vi "Periodic Tasks.vi"(8 "error in":errorcluster) -> ()   [LabVIEW 2020]
doc: "This VI runs in parallel to other tasks. It can contain as many user-defined periodic loops as you need. These can carry out PID or other sorts of timed response."
uses:
  Robot Global Data.vi
  <vilib>/Rock Robotics/Network Tables/NT Write Boolean.vi
  <vilib>/Rock Robotics/Network Tables/NT Write Numeric Array.vi
  <vilib>/Rock Robotics/Network Tables/NT Write Boolean Array.vi
  <vilib>/Rock Robotics/WPI/ThirdParty/Phoenix-LabVIEW/Motor Controller/Controls/CTRE_Phoenix_MotorControl_ControlMode.ctl
  <vilib>/Rock Robotics/WPI/DriverStation/WPI_DriverStationRobotMode2.ctl
  <vilib>/Rock Robotics/Network Tables/NT Write Number.vi
  <vilib>/Rock Robotics/WPI/RobotDrive/WPI_RobotDriveMecanumDrive_Cartesian.vi
  <vilib>/Rock Robotics/WPI/ThirdParty/Phoenix-LabVIEW/Motor Controller/Get/CTRE_Phoenix_MotorController_GetQuadratureData.vi
panel:
  out "Encoder":dbl
  out "Encoder Position":dbl
  out "Slow Speed ON":bool
  out "Backwards ON":bool
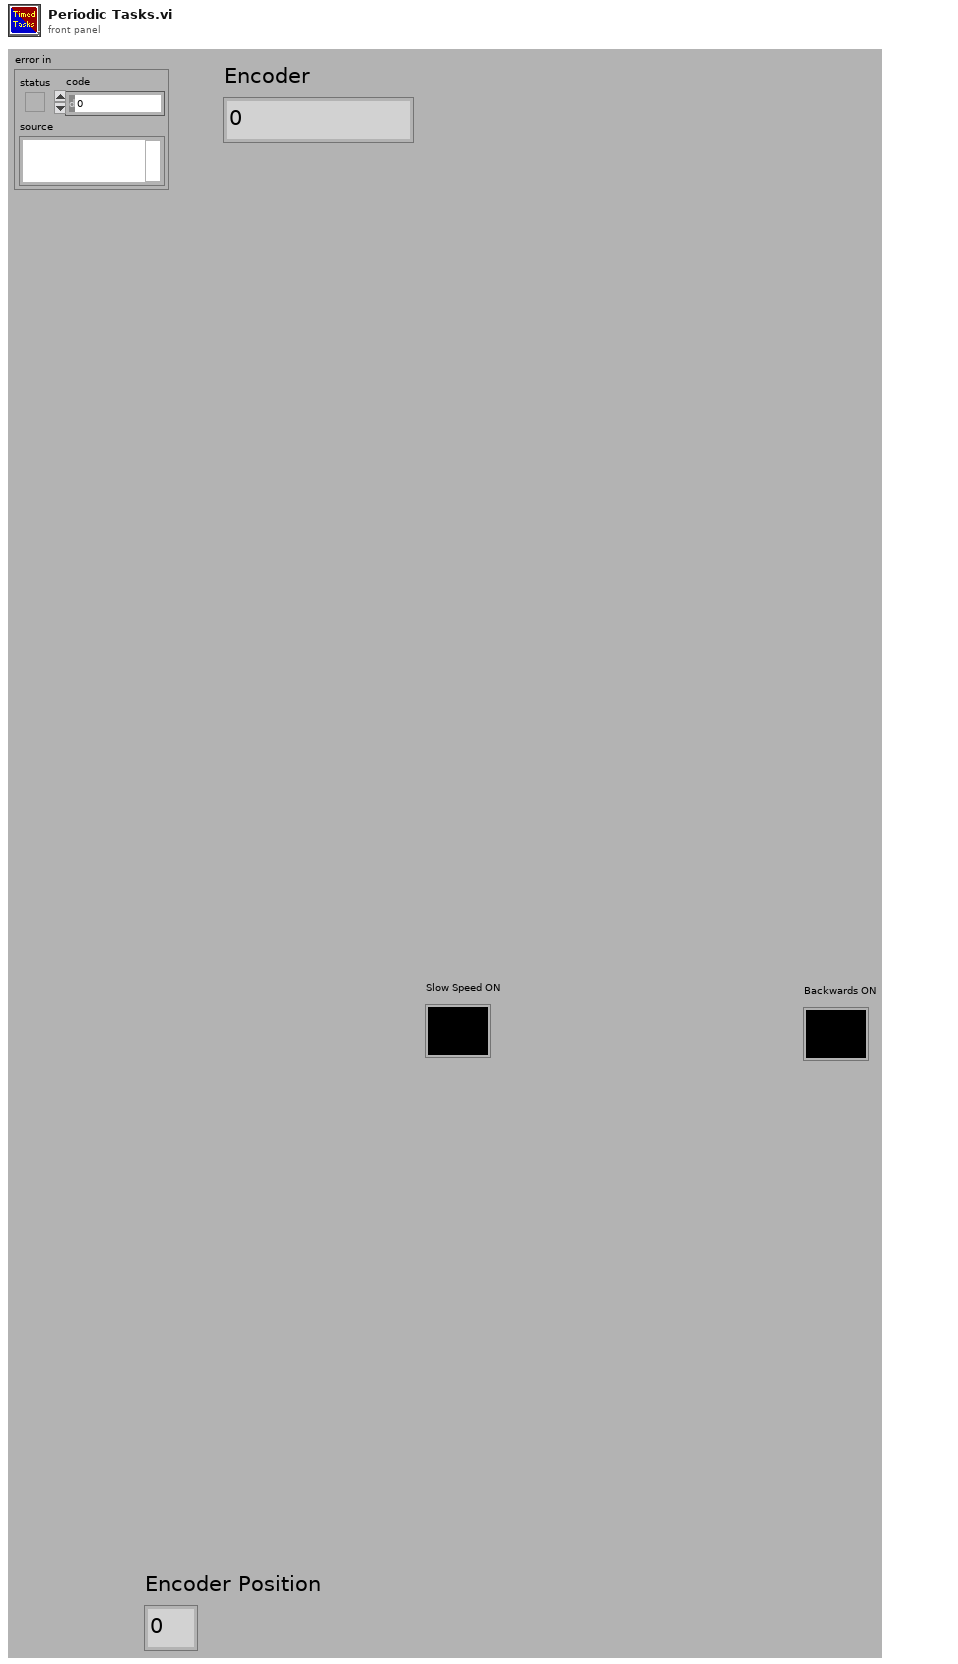
[diagram p1: front panel]
types:
  T1 = typedef "WPI_MotorControlDeviceRef.ctl" = cluster{"DeviceStatus":errorcluster, "Type":T2, "PWM":cluster{"PWM Channel":T3, "DeadBand":T4}, "CAN":cluster{"Device Number":u8, "SetOutput VI Ref":variant, "GetOutput VI Ref":variant, "Enable VI Ref":variant, "Disable VI Ref":variant, "Data":variant}, "Invert":bool, "DIO PWM":cluster{"PWM \"Enable\" Channel":T3, "DIOChannel":T5, "PWM Rate":dbl}}
  T2 = typedef "WPI_MotorControlType.ctl" = enum16{"PWM", "CAN", "DIO PWM"}
  T3 = typedef "FPGA_DIOPWMChannel.ctl" = enum8{"PWM 0", "PWM 1", "PWM 2", "PWM 3", "PWM 4", "PWM 5", "PWM 6", "PWM 7", "PWM 8", "PWM 9", "PWM MXP 0", "PWM MXP 1", "PWM MXP 2", "PWM MXP 3", "PWM MXP 4", "PWM MXP 5", "PWM MXP 6", "PWM MXP 7", "PWM MXP 8", "PWM MXP 9", "Invalid"}
  T4 = typedef "WPI_PWMDeadband.ctl" = cluster{"Name":string, "maxPositivePwm":i32, "minPositivePwm":i32, "centerPwm":i32, "maxNegativePwm":i32, "minNegativePwm":i32, "angularRange":u16}
  T5 = typedef "FPGA_DIOChannel.ctl" = enum8{"DIO 0", "DIO 1", "DIO 2", "DIO 3", "DIO 4", "DIO 5", "DIO 6", "DIO 7", "DIO 8", "DIO 9", "DIO MXP 0", "DIO MXP 1", "DIO MXP 2", "DIO MXP 3", "DIO MXP 4", "DIO MXP 5", "DIO MXP 6", "DIO MXP 7", "DIO MXP 8", "DIO MXP 9", "DIO MXP 10", "DIO MXP 11", "DIO MXP 12", "DIO MXP 13", "DIO MXP 14", "DIO MXP 15", "SPI Port CS1", "SPI Port CS2", "SPI Port CS3", "SPI Port MISO", "SPI Port MOSI", "Invalid"}
  T6 = typedef "WPI_JoystickDevRef.ctl" = cluster{"Device":T7}
  T7 = typedef "WPI_JoystickDeviceEnum.ctl" = enum16{"USB 0", "USB 1", "USB 2", "USB 3", "USB 4", "USB 5"}
  T8 = typedef "WPI_RobotDriveDevRef.ctl" = cluster{"DevStatus":errorcluster, "Motors[]":T1[], "Square Inputs":bool, "Max Output":dbl}
  T9 = typedef "WPI_ServoDeviceRef.ctl" = cluster{"DeviceStatus":errorcluster, "PWM Channel":T3, "DeadBand":T4}
  T10 = typedef "WPI_DriverStationRobotMode2.ctl" = enum16{"Autonomous Disabled", "Autonomous Enabled", "Teleop Disabled", "Teleop Enabled", "Disconnected", "Finish", "Test Disabled", "Test Enabled", "Emergency Stopped"}
  T11 = typedef "CTRE_Phoenix_MotorControl_ControlMode.ctl" = u16
  T12 = typedef "WPI_GyroDevRef.ctl" = cluster{"DevStatus":errorcluster, "Analog Channel":T13, "Gain (VoltsPerDegree/Second)":dbl, "Gyro Type":enum16{"Analog", "XRS450"}, "Handle":i32, "SPI Bus":T14, "Device Found":bool, "Sample Rate":dbl, "Calibrate On Open":bool, "Offset":dbl}
  T13 = typedef "FPGA_AIChannel.ctl" = enum8{"AI 0", "AI 1", "AI 2", "AI 3", "AI MXP 0", "AI MXP 1", "AI MXP 2", "AI MXP 3", "Invalid"}
  T14 = typedef "spi_bus.ctl" = enum16{"SPI On-Board, CS0", "SPI On-Board, CS1", "SPI On-Board, CS2", "SPI On-Board, CS3", "SPI MXP", "Invalid"}
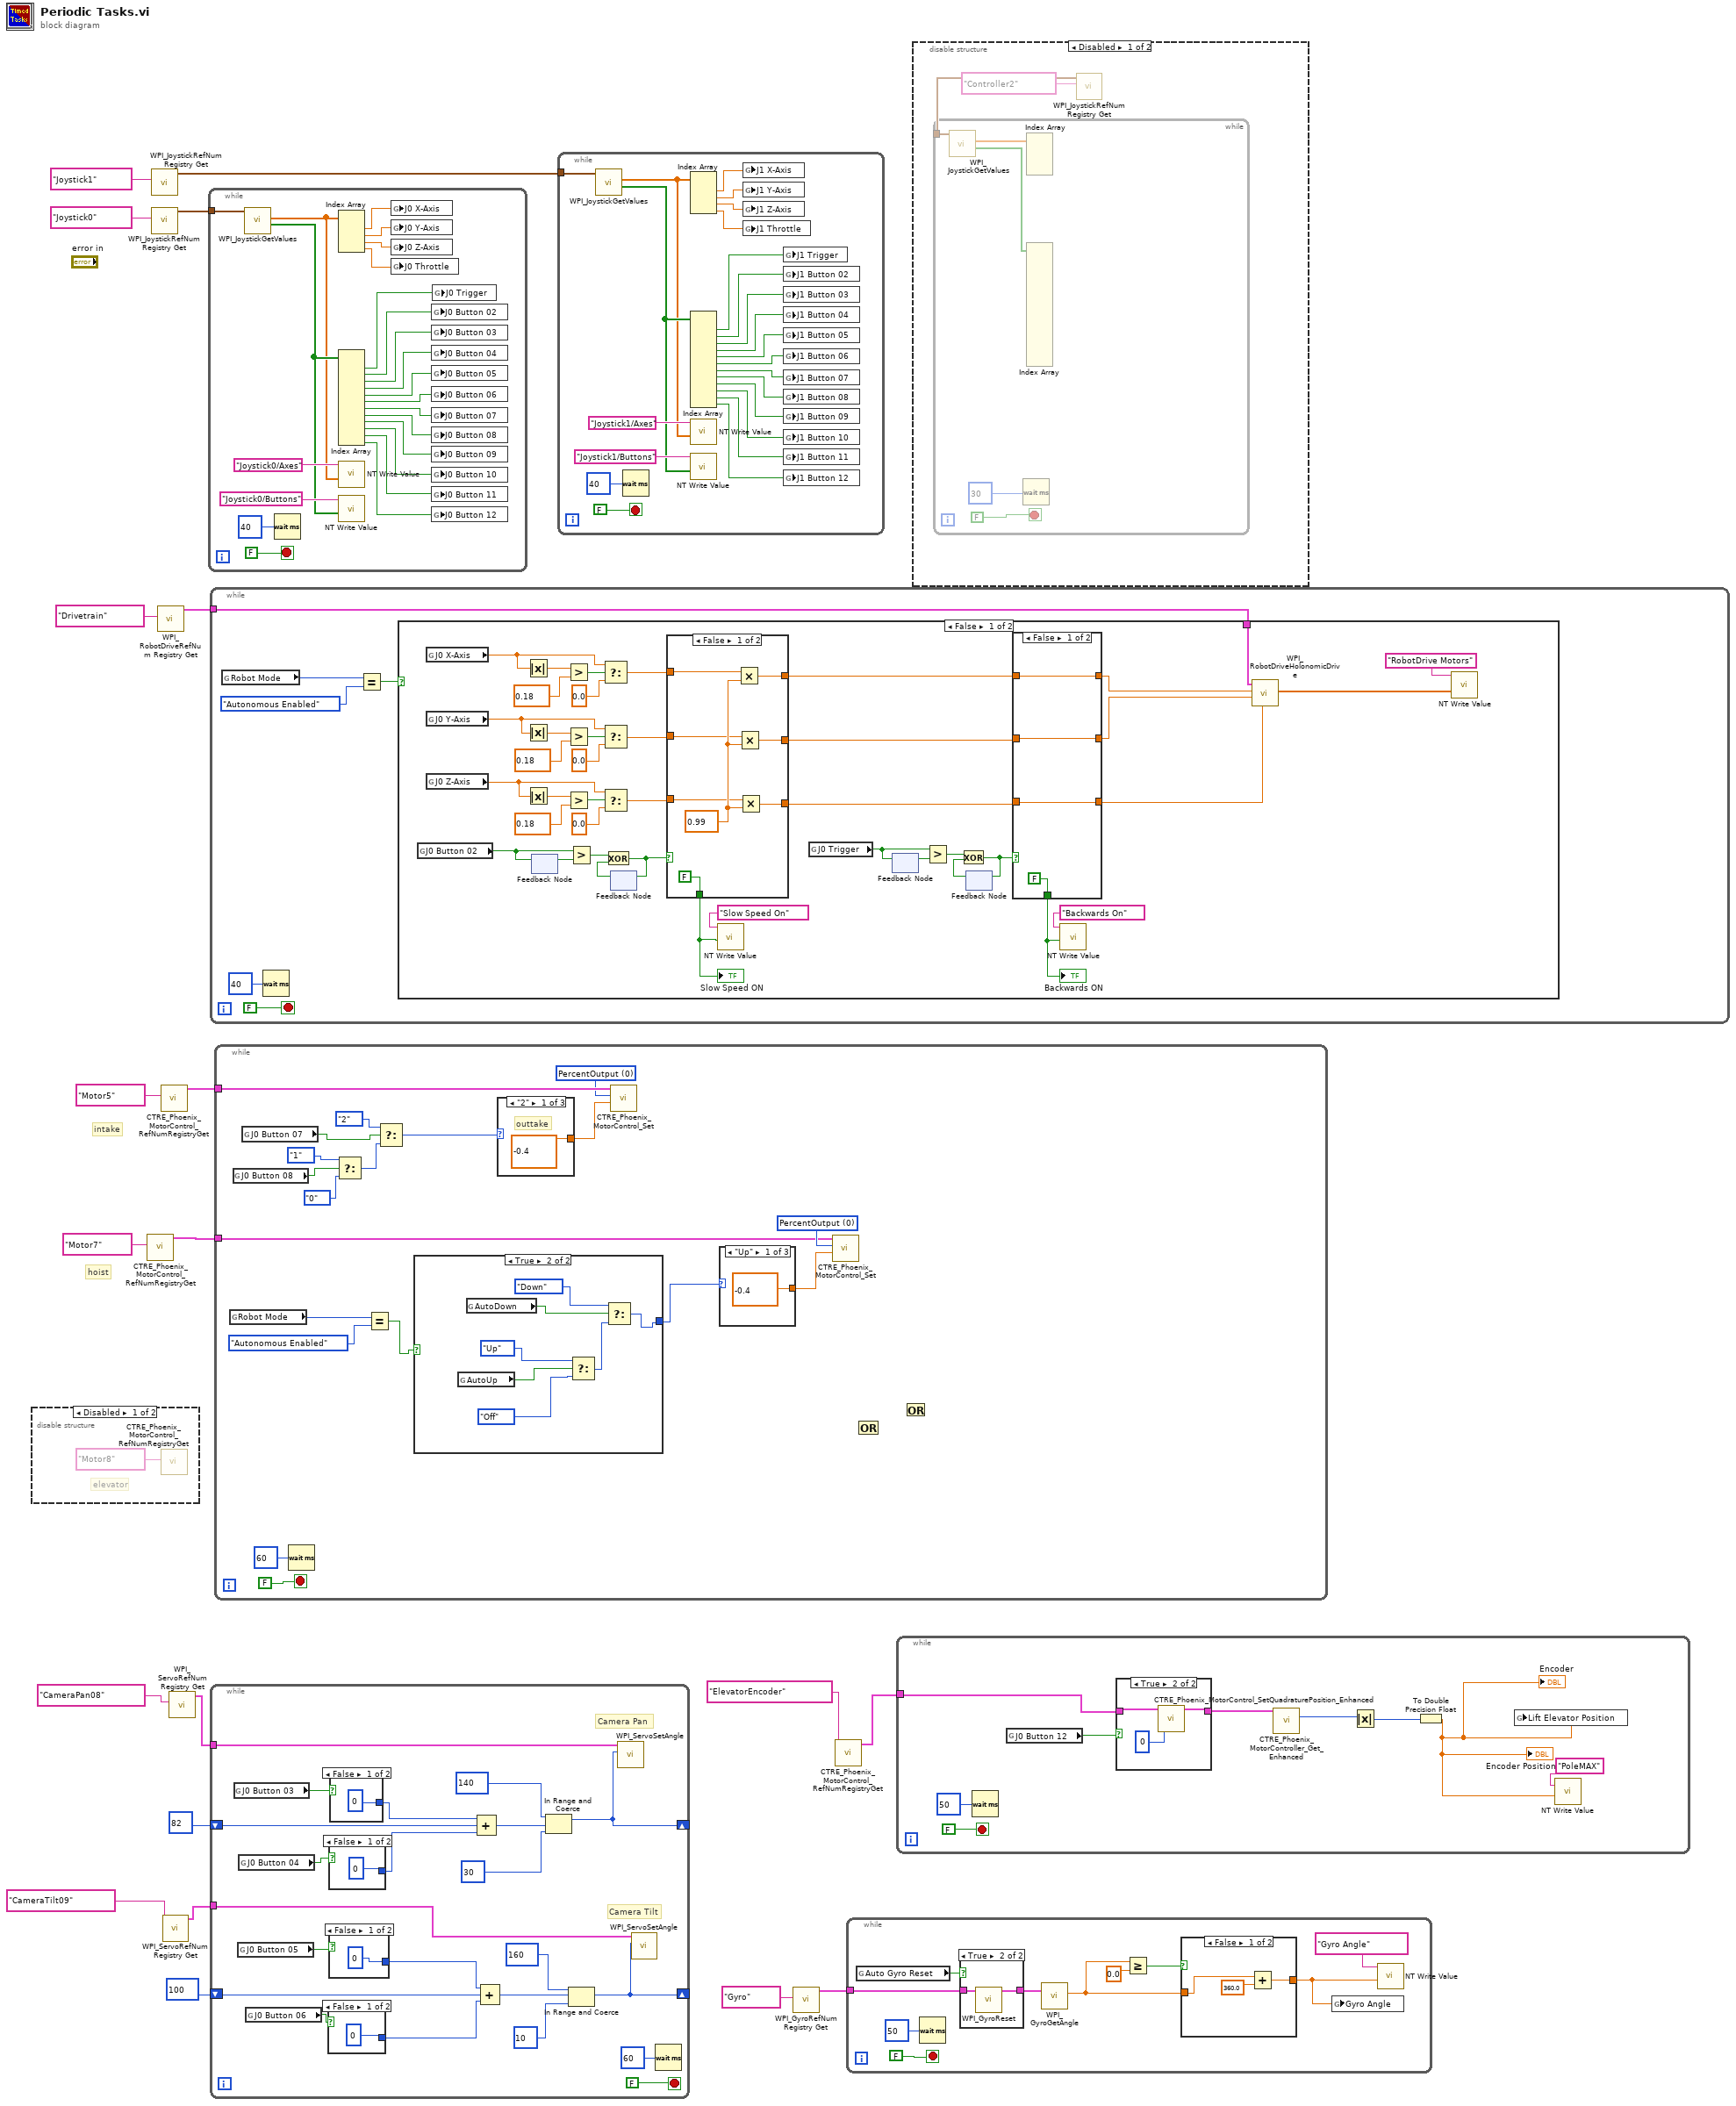
[diagram p0: block diagram]
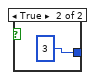
[diagram p6: hidden frame]
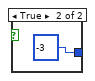
[diagram p7: hidden frame]
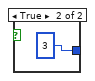
[diagram p8: hidden frame]
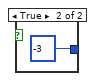
[diagram p9: hidden frame]
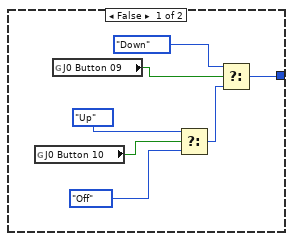
[diagram p11: hidden frame]
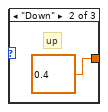
[diagram p12: hidden frame]
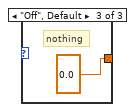
[diagram p13: hidden frame]
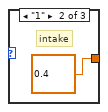
[diagram p14: hidden frame]
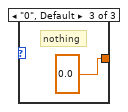
[diagram p15: hidden frame]
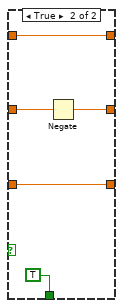
[diagram p16: hidden frame]
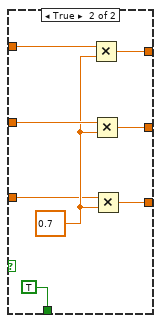
[diagram p17: hidden frame]
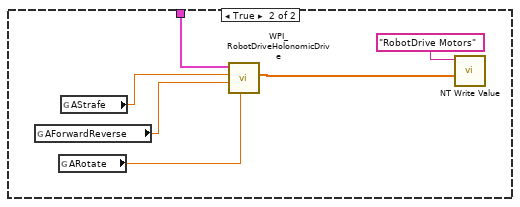
[diagram p18: hidden frame]
diagram:
  # "hoist"
  # "intake"
  n1 = disable-structure shown="Disabled" {
    frame Disabled {
      # "elevator"
      n2 = call <vilib>:"CTRE_Phoenix_MotorControl_RefNumRegistryGet.vi"("refnum name"="Motor8") -> ()  [unwired: 9 in, 2 out]
    }
    frame Enabled {
    }
  }
  n3 = call <vilib>:"CTRE_Phoenix_MotorControl_RefNumRegistryGet.vi"("refnum name"="Motor7") -> ("PhoenixMotorControlDevRef"=w12:T1)  [unwired: 9 in, 1 out]
  n4 = call <vilib>:"WPI_JoystickRefNum Registry Get.vi"("refnum name"="Joystick1") -> ("JoystickDevRef"=w16:T6)  [unwired: 1 in, 9 out]
  n5 = call <vilib>:"WPI_JoystickRefNum Registry Get.vi"("refnum name"="Joystick0") -> ("JoystickDevRef"=w18:T6)  [unwired: 1 in, 9 out]
  n6 = call <vilib>:"WPI_RobotDriveRefNum Registry Get.vi"("refnum name"="Drivetrain") -> ("RobotDriveDevRef"=w3:T8)  [unwired: 9 in, 1 out]
  n7 = call <vilib>:"CTRE_Phoenix_MotorControl_RefNumRegistryGet.vi"("refnum name"="Motor5") -> ("PhoenixMotorControlDevRef"=w13:T1)  [unwired: 9 in, 1 out]
  n8 = call <vilib>:"WPI_ServoRefNum Registry Get.vi"("refnum name"="CameraTilt09") -> ("ServoDeviceRef"=w8:T9)  [unwired: 9 in, 1 out]
  n9 = call <vilib>:"WPI_ServoRefNum Registry Get.vi"("refnum name"="CameraPan08") -> ("ServoDeviceRef"=w9:T9)  [unwired: 9 in, 1 out]
  n10 = while {
    tunnel: w18 -> [w42]
    stop <- FALSE stop-if-true
    n11 = call <vilib>:"WPI_JoystickGetValues.vi"("JoystickDevRef"=w42) -> ("Buttons"=w23:bool[], "Axes"=w22:dbl[])  [unwired: 6 in, 3 out]
    n12 = Wait (ms)(milliseconds to wait=u32 40) -> ()  [unwired: 1 out]
    n13 = Index Array(array=w22) -> (element #1=w41:dbl, element #2=w40:dbl, element #3=w39:dbl, element #4=w38:dbl)  [unwired: 4 in]
    n14 = Index Array(array=w23) -> (element #1=w37:bool, element #2=w36:bool, element #3=w35:bool, element #4=w34:bool, element #5=w33:bool, element #6=w32:bool, element #7=w31:bool, element #8=w30:bool, element #9=w29:bool, element #10=w28:bool, element #11=w27:bool, element #12=w26:bool)  [unwired: 12 in]
    n15 = call-poly <vilib>:"NT Write Value.vi"("Numeric Array"=w22, "Name"="Joystick0/Axes") -> ()  [unwired: 9 in, 1 out]
    n16 = call-poly <vilib>:"NT Write Value.vi"("Boolean Array"=w23, "Name"="Joystick0/Buttons") -> ()  [unwired: 9 in, 1 out]
    n17 = global write "Robot Global Data.vi" "J0 X-Axis"(w41) -> ()
    n18 = global write "Robot Global Data.vi" "J0 Y-Axis"(w40) -> ()
    n19 = global write "Robot Global Data.vi" "J0 Z-Axis"(w39) -> ()
    n20 = global write "Robot Global Data.vi" "J0 Throttle"(w38) -> ()
    n21 = global write "Robot Global Data.vi" "J0 Button 02"(w36) -> ()
    n22 = global write "Robot Global Data.vi" "J0 Button 03"(w35) -> ()
    n23 = global write "Robot Global Data.vi" "J0 Button 04"(w34) -> ()
    n24 = global write "Robot Global Data.vi" "J0 Button 05"(w33) -> ()
    n25 = global write "Robot Global Data.vi" "J0 Button 06"(w32) -> ()
    n26 = global write "Robot Global Data.vi" "J0 Button 07"(w31) -> ()
    n27 = global write "Robot Global Data.vi" "J0 Button 08"(w30) -> ()
    n28 = global write "Robot Global Data.vi" "J0 Button 09"(w29) -> ()
    n29 = global write "Robot Global Data.vi" "J0 Button 10"(w28) -> ()
    n30 = global write "Robot Global Data.vi" "J0 Button 11"(w27) -> ()
    n31 = global write "Robot Global Data.vi" "J0 Button 12"(w26) -> ()
    n32 = global write "Robot Global Data.vi" "J0 Trigger"(w37) -> ()
  }
  n33 = while {
    tunnel: w3 -> [w45]
    stop <- FALSE stop-if-true
    n34 = global read "Robot Global Data.vi" "Robot Mode"() -> (w48:T10)
    n35 = Wait (ms)(milliseconds to wait=u32 40) -> ()  [unwired: 1 out]
    n36 = Equal?(x=w48, y=WPI_DriverStationRobotMode2."Autonomous Enabled" ("Robot Mode")) -> (x = y?=w46:bool)
    n37 = case shown="False" w46 {
      tunnel: w45 -> [w53 w122]
      frame False {
        n38 = global read "Robot Global Data.vi" "J0 Button 02"() -> (w66:bool)
        n39 = global read "Robot Global Data.vi" "J0 X-Axis"() -> (w70:dbl)
        n40 = global read "Robot Global Data.vi" "J0 Y-Axis"() -> (w69:dbl)
        n41 = global read "Robot Global Data.vi" "J0 Z-Axis"() -> (w68:dbl)
        n42 = Absolute Value(x=w70) -> (abs(x)=w85:dbl)
        n43 = Absolute Value(x=w69) -> (abs(x)=w87:dbl)
        n44 = Absolute Value(x=w68) -> (abs(x)=w79:dbl)
        n45 = feedback #1() -> (w90:bool)  [unwired: 1 in]
        n46 = feedback-in #1(w66) -> ()
        n47 = Greater?(x=w85, y=0.18) -> (0:w86:bool)
        n48 = Greater?(x=w87, y=0.18) -> (0:w88:bool)
        n49 = Greater?(x=w79, y=0.18) -> (0:w80:bool)
        n50 = Greater?(x=w66, y=w90) -> (0:w89:bool)
        n51 = Select(t=w70, s=w86, f=0.0) -> (s? t:f=w71:dbl)
        n52 = Select(t=w69, s=w88, f=0.0) -> (s? t:f=w72:dbl)
        n53 = Select(t=w68, s=w80, f=0.0) -> (s? t:f=w73:dbl)
        n54 = feedback #2() -> (w91:bool)  [unwired: 1 in]
        n55 = Exclusive Or(1:w91, 2:w89) -> (0:w67:bool)
        n56 = feedback-in #2(w67) -> ()
        n57 = case shown="False" w67 {
          tunnel: w71 -> [w107 w116]
          tunnel: w72 -> [w106 w115]
          tunnel: [w104 w114] -> w59
          tunnel: [w103 w113] -> w58
          tunnel: w73 -> [w105 w111]
          tunnel: [w102 w110] -> w57
          tunnel: [FALSE ("Boolean") TRUE ("Boolean")] -> w65
          frame False {
            w108 = 0.99 ("y")
            n58 = Multiply(x=w107, y=w108) -> (x*y=w104:dbl)
            n59 = Multiply(x=w106, y=w108) -> (x*y=w103:dbl)
            n60 = Multiply(x=w105, y=w108) -> (x*y=w102:dbl)
          }
          frame True {
            w112 = 0.7 ("y")
            n61 = Multiply(x=w116, y=w112) -> (x*y=w114:dbl)
            n62 = Multiply(x=w115, y=w112) -> (x*y=w113:dbl)
            n63 = Multiply(x=w111, y=w112) -> (x*y=w110:dbl)
          }
        }
        "Slow Speed ON" <- w65
        n64 = call-poly <vilib>:"NT Write Value.vi"("Boolean"=w65, "Name"="Slow Speed On") -> ()  [unwired: 9 in, 1 out]
        n65 = global read "Robot Global Data.vi" "J0 Trigger"() -> (w64:bool)
        n66 = feedback #3() -> (w63:bool)  [unwired: 1 in]
        n67 = feedback-in #3(w64) -> ()
        n68 = Greater?(x=w64, y=w63) -> (0:w74:bool)
        n69 = feedback #4() -> (w62:bool)  [unwired: 1 in]
        n70 = Exclusive Or(1:w62, 2:w74) -> (0:w61:bool)
        n71 = feedback-in #4(w61) -> ()
        n72 = case shown="False" w61 {
          tunnel: w58 -> [w94 w99]
          tunnel: w59 -> [w92 w97]
          tunnel: [w94 w98] -> w55
          tunnel: [w92 w97] -> w54
          tunnel: w57 -> [w93 w96]
          tunnel: [w93 w96] -> w56
          tunnel: [FALSE ("Boolean") TRUE ("Boolean")] -> w60
          frame False {
          }
          frame True {
            n73 = Negate(x=w99) -> (-x=w98:dbl)
          }
        }
        "Backwards ON" <- w60
        n74 = call-poly <vilib>:"NT Write Value.vi"("Boolean"=w60, "Name"="Backwards On") -> ()  [unwired: 9 in, 1 out]
        n75 = call-poly <vilib>:"WPI_RobotDriveHolonomicDrive.vi"("Rotation"=w56, "Y"=w55, "X"=w54, "RobotDriveDevRef"=w53) -> ("Motor Values"=w51:dbl[])  [unwired: 5 in, 2 out]
        n76 = call-poly <vilib>:"NT Write Value.vi"("Numeric Array"=w51, "Name"="RobotDrive Motors") -> ()  [unwired: 9 in, 1 out]
      }
      frame True {
        n77 = global read "Robot Global Data.vi" "AForwardReverse"() -> (w119:dbl)
        n78 = global read "Robot Global Data.vi" "ARotate"() -> (w121:dbl)
        n79 = global read "Robot Global Data.vi" "AStrafe"() -> (w120:dbl)
        n80 = call-poly <vilib>:"WPI_RobotDriveHolonomicDrive.vi"("Rotation"=w121, "Y"=w119, "X"=w120, "RobotDriveDevRef"=w122) -> ("Motor Values"=w118:dbl[])  [unwired: 5 in, 2 out]
        n81 = call-poly <vilib>:"NT Write Value.vi"("Numeric Array"=w118, "Name"="RobotDrive Motors") -> ()  [unwired: 9 in, 1 out]
      }
    }
  }
  n82 = while {
    tunnel: w9 -> [w144]
    tunnel: w8 -> [w143]
    shift-right: [w131] -> _
    shift-left: 82 -> [w124]
    shift-right: [w123] -> _
    shift-left: 100 -> [w140]
    stop <- FALSE stop-if-true
    # "Camera Tilt"
    # "Camera Pan"
    n83 = global read "Robot Global Data.vi" "J0 Button 03"() -> (w127:bool)
    n84 = global read "Robot Global Data.vi" "J0 Button 05"() -> (w129:bool)
    n85 = global read "Robot Global Data.vi" "J0 Button 04"() -> (w128:bool)
    n86 = global read "Robot Global Data.vi" "J0 Button 06"() -> (w130:bool)
    n87 = case shown="False" w130 {
      tunnel: [0 3] -> w139
      frame False {
      }
      frame True {
      }
    }
    n88 = case shown="False" w128 {
      tunnel: [0 3] -> w141
      frame False {
      }
      frame True {
      }
    }
    n89 = case shown="False" w129 {
      tunnel: [0 -3] -> w138
      frame False {
      }
      frame True {
      }
    }
    n90 = case shown="False" w127 {
      tunnel: [0 -3] -> w142
      frame False {
      }
      frame True {
      }
    }
    n91 = Compound Arithmetic op=ADD(w142, w124, w141) -> (w135:i32)
    n92 = Compound Arithmetic op=ADD(w138, w140, w139) -> (w132:i32)
    n93 = In Range and Coerce(upper limit=140, x=w135, lower limit=30) -> (coerced(x)=w131:i32)  [unwired: 1 out]
    n94 = In Range and Coerce(upper limit=160, x=w132, lower limit=10) -> (coerced(x)=w123:i32)  [unwired: 1 out]
    n95 = call <vilib>:"WPI_ServoSetAngle.vi"("Angle"=w131, "ServoDeviceRef"=w144) -> ()  [unwired: 8 in, 2 out]
    n96 = call <vilib>:"WPI_ServoSetAngle.vi"("Angle"=w123, "ServoDeviceRef"=w143) -> ()  [unwired: 8 in, 2 out]
    n97 = Wait (ms)(milliseconds to wait=u32 60) -> ()  [unwired: 1 out]
  }
  n98 = while {
    tunnel: w13 -> [w171]
    tunnel: w12 -> [w157]
    stop <- FALSE stop-if-true
    w160 = T11 0 items=["PercentOutput"=0, "Position"=1, "Velocity"=2, "Current"=3, "Follower"=5, "MotionProfile"=6, "MotionMagic"=7, "MotionProfileArc"=10, "Disabled"=15] ("Control Mode")
    w170 = T11 0 items=["PercentOutput"=0, "Position"=1, "Velocity"=2, "Current"=3, "Follower"=5, "MotionProfile"=6, "MotionMagic"=7, "MotionProfileArc"=10, "Disabled"=15] ("Control Mode")
    n99 = global read "Robot Global Data.vi" "Robot Mode"() -> (w155:T10)
    n100 = global read "Robot Global Data.vi" "J0 Button 08"() -> (w156:bool)
    n101 = global read "Robot Global Data.vi" "J0 Button 07"() -> (w165:bool)
    n102 = Wait (ms)(milliseconds to wait=u32 60) -> ()  [unwired: 1 out]
    n103 = Select(t=enum16{"2", "1", "0", ""}."1", s=w156, f=enum16{"2", "1", "0", ""}."0") -> (s? t:f=w166:enum16{"2", "1", "0", ""})
    n104 = Equal?(x=w155, y=WPI_DriverStationRobotMode2."Autonomous Enabled" ("Robot Mode")) -> (x = y?=w153:bool)
    n105 = Select(t=enum16{"2", "1", "0", ""}."2", s=w165, f=w166) -> (s? t:f=w164:enum16{"2", "1", "0", ""})
    n106 = case shown="True" w153 {
      tunnel: [w176 w179] -> w158
      frame False {
        n107 = global read "Robot Global Data.vi" "J0 Button 10"() -> (w175:bool)
        n108 = global read "Robot Global Data.vi" "J0 Button 09"() -> (w177:bool)
        n109 = Select(t=enum16{"Up", "Down", "Off"}."Up", s=w175, f=enum16{"Up", "Down", "Off"}."Off") -> (s? t:f=w178:enum16{"Up", "Down", "Off"})
        n110 = Select(t=enum16{"Up", "Down", "Off"}."Down", s=w177, f=w178) -> (s? t:f=w176:enum16{"Up", "Down", "Off"})
      }
      frame True {
        n111 = global read "Robot Global Data.vi" "AutoUp"() -> (w185:bool)
        n112 = global read "Robot Global Data.vi" "AutoDown"() -> (w184:bool)
        n113 = Select(t=enum16{"Up", "Down", "Off"}."Up", s=w185, f=enum16{"Up", "Down", "Off"}."Off") -> (s? t:f=w183:enum16{"Up", "Down", "Off"})
        n114 = Select(t=enum16{"Up", "Down", "Off"}."Down", s=w184, f=w183) -> (s? t:f=w179:enum16{"Up", "Down", "Off"})
      }
    }
    n115 = case shown="\"2\"" w164 {
      tunnel: [-0.4 0.4 0.0] -> w169
      frame "2" {
        # "outtake"
      }
      frame "1" {
        # "intake"
      }
      frame "0", Default {
        # "nothing"
      }
    }
    n116 = call <vilib>:"CTRE_Phoenix_MotorControl_Set.vi"("Output"=w169, "Control Mode"=w170, "PhoenixMotorControlDevRef"=w171) -> ()  [unwired: 7 in, 2 out]
    n117 = case shown="\"Up\"" w158 {
      tunnel: [-0.4 0.4 0.0] -> w159
      frame "Up" {
      }
      frame "Down" {
        # "up"
      }
      frame "Off", Default {
        # "nothing"
      }
    }
    n118 = call <vilib>:"CTRE_Phoenix_MotorControl_Set.vi"("Output"=w159, "Control Mode"=w160, "PhoenixMotorControlDevRef"=w157) -> ()  [unwired: 7 in, 2 out]
    n119 = Compound Arithmetic op=OR() -> ()  [unwired: 2 in, 1 out]
    n120 = Or() -> ()  [unwired: 2 in, 1 out]
  }
  n121 = while {
    tunnel: w16 -> [w212]
    stop <- FALSE stop-if-true
    n122 = call <vilib>:"WPI_JoystickGetValues.vi"("JoystickDevRef"=w212) -> ("Buttons"=w193:bool[], "Axes"=w192:dbl[])  [unwired: 6 in, 3 out]
    n123 = Wait (ms)(milliseconds to wait=u32 40) -> ()  [unwired: 1 out]
    n124 = Index Array(array=w192) -> (element #1=w211:dbl, element #2=w210:dbl, element #3=w209:dbl, element #4=w208:dbl)  [unwired: 4 in]
    n125 = Index Array(array=w193) -> (element #1=w207:bool, element #2=w206:bool, element #3=w205:bool, element #4=w204:bool, element #5=w203:bool, element #6=w202:bool, element #7=w201:bool, element #8=w200:bool, element #9=w199:bool, element #10=w198:bool, element #11=w197:bool, element #12=w196:bool)  [unwired: 12 in]
    n126 = call-poly <vilib>:"NT Write Value.vi"("Numeric Array"=w192, "Name"="Joystick1/Axes") -> ()  [unwired: 9 in, 1 out]
    n127 = call-poly <vilib>:"NT Write Value.vi"("Boolean Array"=w193, "Name"="Joystick1/Buttons") -> ()  [unwired: 9 in, 1 out]
    n128 = global write "Robot Global Data.vi" "J1 X-Axis"(w211) -> ()
    n129 = global write "Robot Global Data.vi" "J1 Y-Axis"(w210) -> ()
    n130 = global write "Robot Global Data.vi" "J1 Z-Axis"(w209) -> ()
    n131 = global write "Robot Global Data.vi" "J1 Throttle"(w208) -> ()
    n132 = global write "Robot Global Data.vi" "J1 Trigger"(w207) -> ()
    n133 = global write "Robot Global Data.vi" "J1 Button 02"(w206) -> ()
    n134 = global write "Robot Global Data.vi" "J1 Button 03"(w205) -> ()
    n135 = global write "Robot Global Data.vi" "J1 Button 04"(w204) -> ()
    n136 = global write "Robot Global Data.vi" "J1 Button 05"(w203) -> ()
    n137 = global write "Robot Global Data.vi" "J1 Button 06"(w202) -> ()
    n138 = global write "Robot Global Data.vi" "J1 Button 07"(w201) -> ()
    n139 = global write "Robot Global Data.vi" "J1 Button 08"(w200) -> ()
    n140 = global write "Robot Global Data.vi" "J1 Button 09"(w199) -> ()
    n141 = global write "Robot Global Data.vi" "J1 Button 10"(w198) -> ()
    n142 = global write "Robot Global Data.vi" "J1 Button 11"(w197) -> ()
    n143 = global write "Robot Global Data.vi" "J1 Button 12"(w196) -> ()
  }
  n144 = call <vilib>:"WPI_GyroRefNum Registry Get.vi"("refnum name"="Gyro") -> ("GyroDevRef"=w6:T12)  [unwired: 9 in, 1 out]
  n145 = call <vilib>:"CTRE_Phoenix_MotorControl_RefNumRegistryGet.vi"("refnum name"="ElevatorEncoder") -> ("PhoenixMotorControlDevRef"=w1:T1)  [unwired: 9 in, 1 out]
  n146 = while {
    tunnel: w6 -> [w224]
    stop <- FALSE stop-if-true
    n147 = global read "Robot Global Data.vi" "Auto Gyro Reset"() -> (w222:bool)
    n148 = Wait (ms)(milliseconds to wait=u32 50) -> ()  [unwired: 1 out]
    n149 = case shown="True" w222 {
      tunnel: w224 -> [w229 w231]
      tunnel: [w229 w230] -> w223
      frame False {
      }
      frame True {
        n150 = call <vilib>:"WPI_GyroReset.vi"("GyroDevRef"=w231) -> ("GyroDevRef"=w230:T12)  [unwired: 9 in, 1 out]
      }
    }
    n151 = call <vilib>:"WPI_GyroGetAngle.vi"("GyroDevRef"=w223) -> ("Angle"=w219:dbl)  [unwired: 6 in, 4 out]
    n152 = Greater Or Equal?(x=w219, y=0.0) -> (x >= y?=w217:bool)
    n153 = case shown="False" w217 {
      tunnel: w219 -> [w226 w228]
      tunnel: [w225 w228] -> w215
      frame False {
        n154 = Add(x=w226, y=360.0) -> (x+y=w225:dbl)
      }
      frame True {
      }
    }
    n155 = global write "Robot Global Data.vi" "Gyro Angle"(w215) -> ()
    n156 = call-poly <vilib>:"NT Write Value.vi"("Numeric"=w215, "Name"="Gyro Angle" ("refnum name")) -> ()  [unwired: 9 in, 1 out]
  }
  n157 = while {
    tunnel: w1 -> [w238]
    stop <- FALSE stop-if-true
    n158 = Wait (ms)(milliseconds to wait=u32 50) -> ()  [unwired: 1 out]
    n159 = global read "Robot Global Data.vi" "J0 Button 12"() -> (w237:bool)
    n160 = case shown="True" w237 {
      tunnel: [w241 w243] -> w236
      tunnel: w238 -> [w241 w242]
      frame False {
      }
      frame True {
        n161 = call <vilib>:"CTRE_Phoenix_MotorControl_SetQuadraturePosition_Enhanced.vi"("New Position"=0, "PhoenixMotorControlDevRef"=w242) -> ("PhoenixMotorControlDevRef"=w243:T1)  [unwired: 8 in, 1 out]
      }
    }
    n162 = call-poly <vilib>:"CTRE_Phoenix_MotorController_Get_Enhanced.vi"("PhoenixMotorControlDevRef"=w236) -> ("Quadrature Position"=w235:i32)  [unwired: 11 in, 3 out]
    n163 = Absolute Value(x=w235) -> (abs(x)=w234:i32)
    n164 = To Double Precision Float(number=w234) -> (double precision float=w232:dbl)
    "Encoder Position" <- w232
    "Encoder" <- w232
    n165 = global write "Robot Global Data.vi" "Lift Elevator Position"(w232) -> ()
    n166 = call-poly <vilib>:"NT Write Value.vi"("Numeric"=w232, "Name"="PoleMAX") -> ()  [unwired: 9 in, 1 out]
  }
  n167 = disable-structure shown="Disabled" {
    frame Disabled {
      n168 = call <vilib>:"WPI_JoystickRefNum Registry Get.vi"("refnum name"="Controller2") -> ("JoystickDevRef"=w245:T6)  [unwired: 1 in, 9 out]
      n169 = while {
        tunnel: w245 -> [w251]
        stop <- FALSE stop-if-true
        n170 = call <vilib>:"WPI_JoystickGetValues.vi"("JoystickDevRef"=w251) -> ("Buttons"=w247:bool[], "Axes"=w248:dbl[])  [unwired: 6 in, 3 out]
        n171 = Wait (ms)(milliseconds to wait=u32 30) -> ()  [unwired: 1 out]
        n172 = Index Array(array=w248) -> ()  [unwired: 4 in, 4 out]
        n173 = Index Array(array=w247) -> ()  [unwired: 16 in, 16 out]
      }
    }
    frame Enabled {
    }
  }
